vi "Time Unflatten.vi"() -> ()   [LabVIEW 2017]
panel:
  in  "Boolean":bool
  in  "String 2":string
  out "count":u32
  out "x-y":u32
  in  "String":string
  # "String to array of bytes to index is five times faster than typecast,\n25 times faster than unflatten"
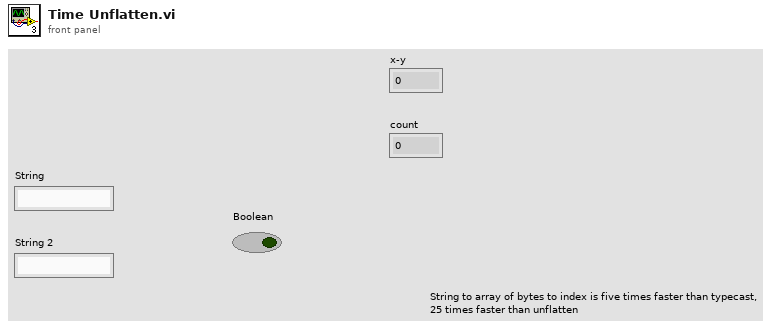
[diagram p1: front panel]
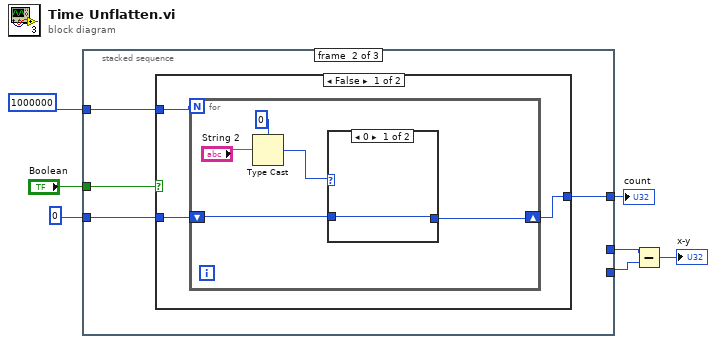
[diagram p0: block diagram]
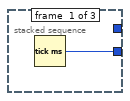
[diagram p2: hidden frame]
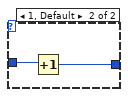
[diagram p3: hidden frame]
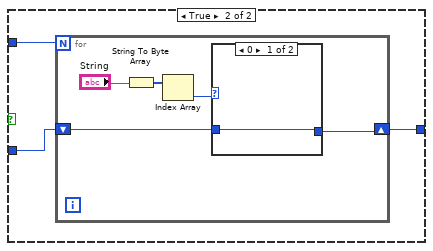
[diagram p4: hidden frame]
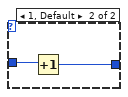
[diagram p5: hidden frame]
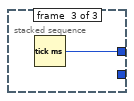
[diagram p6: hidden frame]
diagram:
  n1 = stacked-sequence {
    tunnel: [w8 _ _] -> w6
    tunnel: [_ _ w35] -> w7
    tunnel: [_ w12 _] -> w4
    tunnel: 1000000 -> [_ w11 _]
    tunnel: "Boolean" -> [_ w10 _]
    tunnel: 0 -> [_ w9 _]
    frame #0 {
      n2 = Tick Count (ms)() -> (millisecond timer value=w8:u32)
    }
    frame #1 {
      n3 = case shown="False" w10 {
        tunnel: [w13 w26] -> w12
        tunnel: w11 -> [w15 w25]
        tunnel: w9 -> [w14 w24]
        frame False {
          n4 = for {
            N: w15 -> [_]
            shift-right: [w19] -> w13
            shift-left: w14 -> [w20]
            n5 = Type Cast(type=u8 0, x="String 2") -> (*(type *) &x=w16:u8)
            n6 = case shown="0" w16 {
              tunnel: w20 -> [w21 w23]
              tunnel: [w21 w22] -> w19
              frame 0 {
              }
              frame 1, Default {
                n7 = Increment(x=w23) -> (x+1=w22:i32)
              }
            }
          }
        }
        frame True {
          n8 = for {
            N: w25 -> [_]
            shift-right: [w28] -> w26
            shift-left: w24 -> [w29]
            n9 = String To Byte Array(string="String") -> (unsigned byte array=w31:u8[])
            n10 = Index Array(array=w31) -> (element=w30:u8)  [unwired: 1 in]
            n11 = case shown="0" w30 {
              tunnel: w29 -> [w32 w34]
              tunnel: [w32 w33] -> w28
              frame 0 {
              }
              frame 1, Default {
                n12 = Increment(x=w34) -> (x+1=w33:i32)
              }
            }
          }
        }
      }
    }
    frame #2 {
      n13 = Tick Count (ms)() -> (millisecond timer value=w35:u32)
    }
  }
  "count" <- w4
  n14 = Subtract(x=w7, y=w6) -> (x-y=→"x-y":u32)
